vi "Popup_SpikeThreshold.vi"(8 "에러 입력(에러 없음)":errorcluster, 10 "Threshold (mV)":dbl, 11 "Caller VI Reference":refnum<vi>) -> (0 "에러 출력":errorcluster, 3 "Threshold (mV) OUT":dbl)   [LabVIEW 2017]
panel:
  in  "OK":bool
  # "Enter threshold to detect spikes"
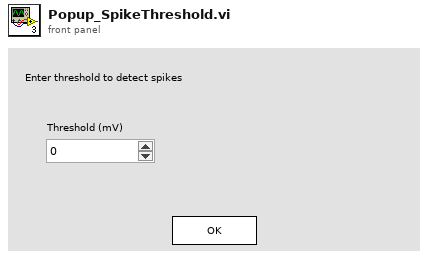
[diagram p1: front panel]
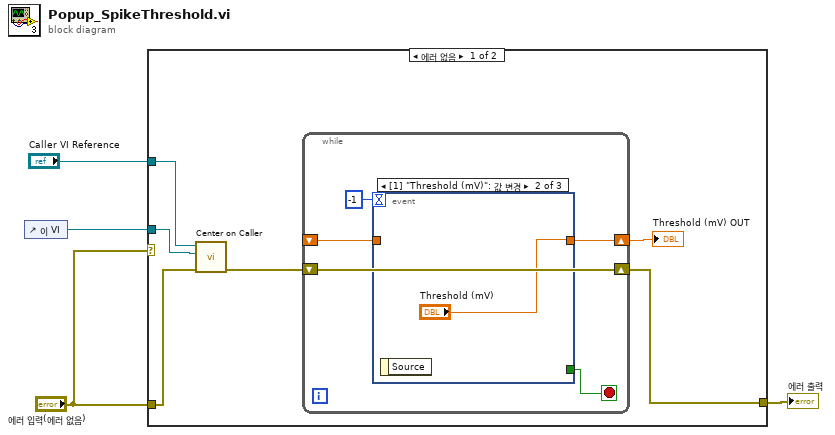
[diagram p0: block diagram]
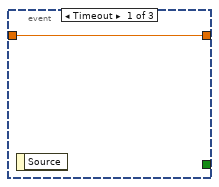
[diagram p2: hidden frame]
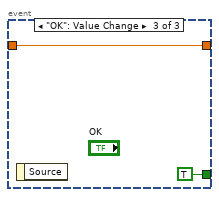
[diagram p3: hidden frame]
diagram:
  n1 = control-ref of="이 VI"() -> (w1:refnum<vi>)
  n2 = case shown="에러 없음" "에러 입력(에러 없음)" {
    tunnel: "Caller VI Reference" -> [w9 _]
    tunnel: "에러 입력(에러 없음)" -> [w8 w20]
    tunnel: [w6 w20] -> w2
    tunnel: w1 -> [w5 _]
    frame No Error {
      n3 = call <userlib>:"Center on Caller.vi"("에러 입력(에러 없음)"=w8, "Child VI Reference"=w5, "Caller VI Reference"=w9) -> ("에러 출력"=w7:errorcluster)  [unwired: 8 in]
      n4 = while {
        shift-right: [w15] -> w10
        shift-left: _ -> [w13]
        shift-right: [w11] -> w6
        shift-left: w7 -> [w11]
        stop <- w14 stop-if-true
        n5 = event shown="[1] \"Threshold (mV)\": 값 변경" {
          selector: _ -> [_ _ _]
          dyn-events: _ -> [_ _ _]
          timeout: -1 -> [_ _ _]
          tunnel: [w16 "Threshold (mV)" w18] -> w15
          tunnel: [_ _ TRUE] -> w14
          tunnel: w13 -> [w16 _ w18]
          event Timeout {
            n6 = event-data() -> ()  [unwired: 1 in, 1 out]
          }
          event "Threshold (mV)": Value Change {
            n7 = event-data() -> ()  [unwired: 1 in, 1 out]
          }
          event "OK": Value Change {
            n8 = event-data() -> ()  [unwired: 1 in, 1 out]
          }
        }
      }
      "Threshold (mV) OUT" <- w10
    }
    frame Error {
    }
  }
  "에러 출력" <- w2
